vi "Current_Rotary_Speed.vi"(10 "Number Of Rotations prev":dbl, 11 "Number Of Rotations":dbl) -> (3 "Current Rotary Speed":dbl)   [LabVIEW 2018]
doc: "This VI calculates current rotary speed in radians per second. It does so by checking whether current number of rotations isn't equal to previous number of rotations and if the wheel is spinning, it calculates the change in number of rotations, multiplies it by 2Pi and divides it by change in time (0.1 s).\n\nInputs:\nNumber of rotations;\nNumber of rotations prev.\n\nOutputs:\nCurrent rotary speed."
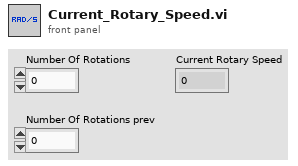
[diagram p1: front panel]
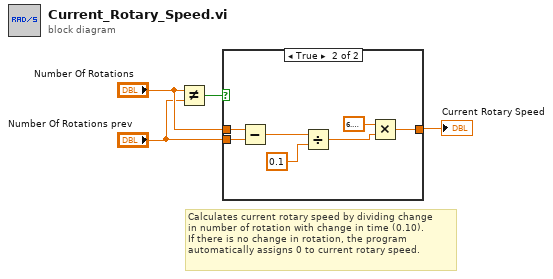
[diagram p0: block diagram]
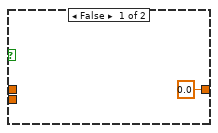
[diagram p2: hidden frame]
diagram:
  # "Calculates current rotary speed by dividing change\nin number of rotation with change in time (0.10).\nIf there is no change in rotation, the program\nautomatically assigns 0 to current rotary speed."
  n1 = Not Equal?(x="Number Of Rotations", y="Number Of Rotations prev") -> (x != y?=w3:bool)
  n2 = case shown="True" w3 {
    tunnel: [0.0 w11] -> w4
    tunnel: "Number Of Rotations prev" -> [_ w10]
    tunnel: "Number Of Rotations" -> [_ w9]
    frame False {
    }
    frame True {
      n3 = Subtract(x=w9, y=w10) -> (x-y=w8:dbl)
      n4 = Divide(x=w8, y=0.1) -> (x/y=w7:dbl)
      n5 = Multiply(x=6.283185307179586, y=w7) -> (x*y=w11:dbl)
    }
  }
  "Current Rotary Speed" <- w4
